vi "Distance to RPM_V1.vi"(3 "Personality":string, 4 "Target Distance":dbl) -> (1 "Shooter RPM Control":dbl)   [LabVIEW 2011]
uses:
  Robot Global Data.vi
panel:
  out "Shooter RPM Offset":dbl
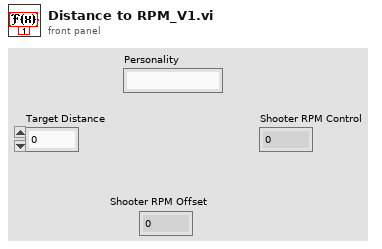
[diagram p1: front panel]
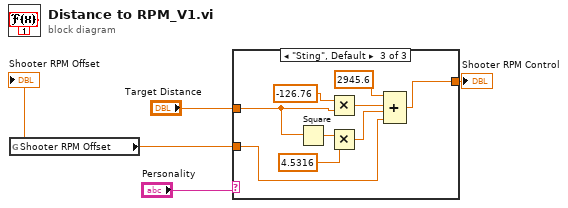
[diagram p0: block diagram]
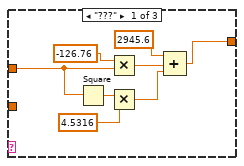
[diagram p2: hidden frame]
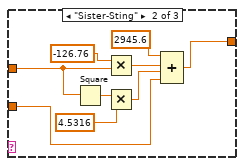
[diagram p3: hidden frame]
diagram:
  n1 = global read "Robot Global Data.vi" "Shooter RPM Offset"() -> (w1:dbl)
  "Shooter RPM Offset" <- w1
  n2 = case shown="\"Sting\", Default" "Personality" {
    tunnel: [w6 w15 w27] -> w3
    tunnel: "Target Distance" -> [w5 w14 w23]
    tunnel: w1 -> [_ w13 w22]
    frame "???" {
      n3 = Square(x=w5) -> (x^2=w7:dbl)
      n4 = Multiply(x=-126.76, y=w5) -> (x*y=w10:dbl)
      n5 = Multiply(x=w7, y=4.5316) -> (x*y=w11:dbl)
      n6 = Compound Arithmetic op=ADD(2945.6 ("value"), w10, w11) -> (w6:dbl)
    }
    frame "Sister-Sting" {
      n7 = Square(x=w14) -> (x^2=w21:dbl)
      n8 = Multiply(x=-126.76, y=w14) -> (x*y=w18:dbl)
      n9 = Multiply(x=w21, y=4.5316) -> (x*y=w17:dbl)
      n10 = Compound Arithmetic op=ADD(2945.6 ("value"), w18, w17, w13) -> (w15:dbl)
    }
    frame "Sting", Default {
      n11 = Square(x=w23) -> (x^2=w30:dbl)
      n12 = Multiply(x=-126.76, y=w23) -> (x*y=w26:dbl)
      n13 = Multiply(x=w30, y=4.5316) -> (x*y=w25:dbl)
      n14 = Compound Arithmetic op=ADD(2945.6 ("value"), w26, w25, w22) -> (w27:dbl)
    }
  }
  "Shooter RPM Control" <- w3
